vi "scale_3_element_find_peak.vi"(11 "2D array in":dbl[][](array[numeric])=[[5.0, 5.0, 5.0], [0.0, 5.0, 5.0], [5.0, 5.0, 5.0]]) -> (2 "y offset":dbl, 3 "x offset":dbl)   [LabVIEW 2010]
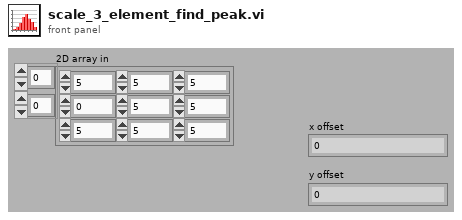
[diagram p1: front panel]
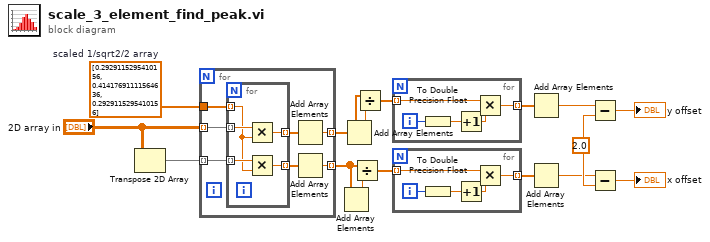
[diagram p0: block diagram]
diagram:
  w3 = 2.0 ("y")
  w13 = dbl[] [0.2929115295410156, 0.41417691111564636, 0.2929115295410156]  # scaled 1/sqrt2/2 array
  n1 = Transpose 2D Array(2D array="2D array in") -> (transposed array=w16:dbl[][])
  n2 = for {
    tunnel: w16 -> [w22] mode=indexing
    tunnel: [w21] -> w14 mode=indexing
    tunnel: w13 -> [w23]
    tunnel: "2D array in" -> [w19] mode=indexing
    tunnel: [w17] -> w9 mode=indexing
    n3 = for {
      tunnel: [w27] -> w20 mode=indexing
      tunnel: w23 -> [w25] mode=indexing
      tunnel: w22 -> [w28] mode=indexing
      tunnel: w19 -> [w26] mode=indexing
      tunnel: [w24] -> w18 mode=indexing
      n4 = Multiply(x=w26, y=w25) -> (x*y=w24:dbl)
      n5 = Multiply(x=w28, y=w25) -> (x*y=w27:dbl)
    }
    n6 = Add Array Elements(numeric array=w18) -> (sum=w17:dbl)
    n7 = Add Array Elements(numeric array=w20) -> (sum=w21:dbl)
  }
  n8 = Add Array Elements(numeric array=w14) -> (sum=w15:dbl)
  n9 = Add Array Elements(numeric array=w9) -> (sum=w10:dbl)
  n10 = Divide(x=w14, y=w15) -> (x/y=w8:dbl[])
  n11 = Divide(x=w9, y=w10) -> (x/y=w11:dbl[])
  n12 = for {
    tunnel: w11 -> [w33] mode=indexing
    tunnel: [w31] -> w12 mode=indexing
    i -> [w32]
    n13 = To Double Precision Float(number=w32) -> (double precision float=w29:dbl)
    n14 = Increment(x=w29) -> (x+1=w30:dbl)
    n15 = Multiply(x=w33, y=w30) -> (x*y=w31:dbl)
  }
  n16 = for {
    tunnel: w8 -> [w38] mode=indexing
    tunnel: [w36] -> w7 mode=indexing
    i -> [w37]
    n17 = To Double Precision Float(number=w37) -> (double precision float=w34:dbl)
    n18 = Increment(x=w34) -> (x+1=w35:dbl)
    n19 = Multiply(x=w38, y=w35) -> (x*y=w36:dbl)
  }
  n20 = Add Array Elements(numeric array=w12) -> (sum=w5:dbl)
  n21 = Add Array Elements(numeric array=w7) -> (sum=w2:dbl)
  n22 = Subtract(x=w5, y=w3) -> (x-y=→"y offset":dbl)
  n23 = Subtract(x=w2, y=w3) -> (x-y=→"x offset":dbl)
